vi "niDTS WLAN OFDM Rx Test UTIL OFDM Parameters to WLAN Rx Parameters.vi"(7 "WLAN Rx Input Parameters":T1={"OFDM Data Rate (Mbps)"=enum."6", "Chains"=[TRUE, FALSE, FALSE, FALSE], "Bandwidth (Hz)"=enum."20 MHz", "Channel"=0, "Power (dBm)"=1.0, "16 symbols"=TRUE, "Payload Length (bytes)"=0, "Idle Interval (s)"=7.0, "External Attenuation (dB)"=[0.0, 0.0, 0.0, 0.0], "RX Measurement Parameters"={"Number of Packets"=1000, "MacAddress"="FF:FF:FF:FF:FF:FF"}} {"Idle Interval (s)" format="%_3p"}) -> (8 "WLAN Tx Parameters":T5={"Standard"=enum."802.11 n HT", "DSSS Data Rate (Mbps)"=enum."1", "OFDM Data Rate (Mbps)"=enum."54", "MCS Index"=7, "N Spatial Streams"=1, "Chains"=[TRUE, FALSE, FALSE, FALSE], "Bandwidth (Hz)"=enum."20 MHz", "Channel"=1, "Power (dBm)"=0.0, "Guard Interval"=enum."SHORT", "FEC Coding"=enum."LDPC", "16 symbols"=TRUE, "Payload Length (bytes)"=1500, "Idle Interval (s)"=0.0001, "External Attenuation (dB)"=[0.0, 0.0, 0.0, 0.0], "RX Measurement Parameters"={"Number of Packets"=1000, "MacAddress"="FF:FF:FF:FF:FF:FF"}} {"Idle Interval (s)" format="%_3p"})   [LabVIEW 2014, in "niDTS WLAN.lvlib"]
uses:
  niDTS WLAN.lvlib
  Rx Test/Includes/niDTS WLAN Rx Test INC Parameters.ctl
  Includes/niDTS WLAN INC Standard.ctl
  Includes/niDTS WLAN INC DSSS Data Rate.ctl
  Includes/niDTS WLAN INC OFDM Data Rate.ctl
  Includes/niDTS WLAN INC CH BW.ctl
  Includes/niDTS WLAN INC GI.ctl
  Includes/niDTS WLAN INC FEC Coding.ctl
  Rx Test/Includes/niDTS WLAN INC RX Measurement Parameters.ctl
  Includes/niDTS WLAN Rx Test INC OFDM Parameters.ctl
  Includes/niDTS WLAN INC CH BW DSSS.ctl
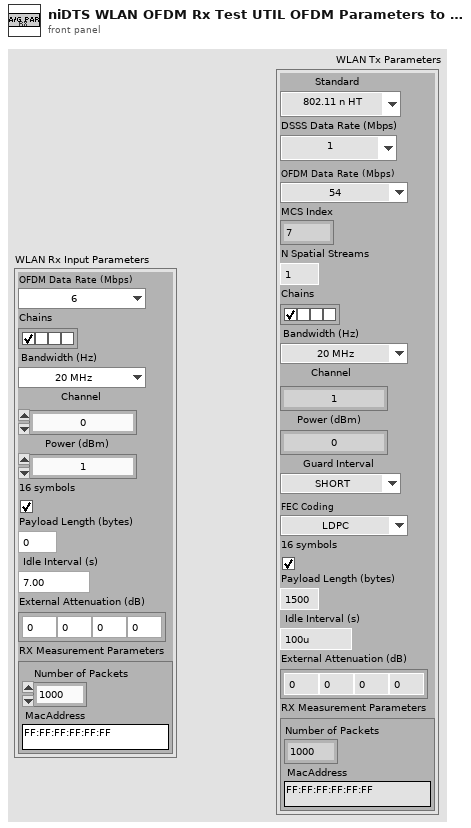
[diagram p1: front panel]
types:
  T1 = typedef "niDTS WLAN.lvlib/niDTS WLAN Rx Test INC OFDM Parameters.ctl" = cluster{"OFDM Data Rate (Mbps)":T2, "Chains":bool[], "Bandwidth (Hz)":T3, "Channel":i32, "Power (dBm)":dbl, "16 symbols":bool, "Payload Length (bytes)":i32, "Idle Interval (s)":dbl, "External Attenuation (dB)":dbl[], "RX Measurement Parameters":T4}
  T2 = typedef "niDTS WLAN.lvlib/niDTS WLAN INC OFDM Data Rate.ctl" = enum16{"6", "9", "12", "18", "24", "36", "48", "54"}
  T3 = typedef "niDTS WLAN.lvlib/niDTS WLAN INC CH BW DSSS.ctl" = enum16{"20 MHz"}
  T4 = typedef "niDTS WLAN.lvlib/niDTS WLAN INC RX Measurement Parameters.ctl" = cluster{"Number of Packets":i32, "MacAddress":string}
  T5 = typedef "niDTS WLAN.lvlib/niDTS WLAN Rx Test INC Parameters.ctl" = cluster{"Standard":T6, "DSSS Data Rate (Mbps)":T7, "OFDM Data Rate (Mbps)":T2, "MCS Index":i32, "N Spatial Streams":i32, "Chains":bool[], "Bandwidth (Hz)":T8, "Channel":i32, "Power (dBm)":dbl, "Guard Interval":T9, "FEC Coding":T10, "16 symbols":bool, "Payload Length (bytes)":i32, "Idle Interval (s)":dbl, "External Attenuation (dB)":dbl[], "RX Measurement Parameters":T4}
  T6 = typedef "niDTS WLAN.lvlib/niDTS WLAN INC Standard.ctl" = enum16{"802.11 b DSSS", "802.11 a/g OFDM", "802.11 n HT", "802.11 ac VHT"}
  T7 = typedef "niDTS WLAN.lvlib/niDTS WLAN INC DSSS Data Rate.ctl" = enum16{"1", "2", "5.5", "11"}
  T8 = typedef "niDTS WLAN.lvlib/niDTS WLAN INC CH BW.ctl" = enum16{"20 MHz", "40 MHz", "80 MHz", "160 MHz"}
  T9 = typedef "niDTS WLAN.lvlib/niDTS WLAN INC GI.ctl" = enum16{"LONG", "SHORT"}
  T10 = typedef "niDTS WLAN.lvlib/niDTS WLAN INC FEC Coding.ctl" = enum16{"BCC", "LDPC"}
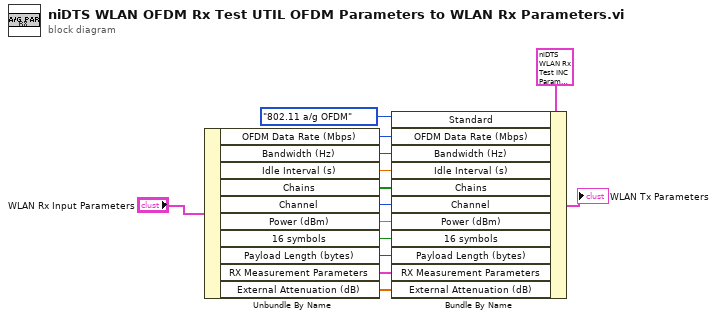
[diagram p0: block diagram]
diagram:
  n1 = Unbundle By Name("WLAN Rx Input Parameters") -> ("OFDM Data Rate (Mbps)"=w11:T2, "Bandwidth (Hz)"=w10:T3, "Idle Interval (s)"=w9:dbl, "Chains"=w8:bool[], "Channel"=w7:i32, "Power (dBm)"=w6:dbl, "16 symbols"=w5:bool, "Payload Length (bytes)"=w4:i32, "RX Measurement Parameters"=w3:T4, "External Attenuation (dB)"=w1:dbl[])
  n2 = Bundle By Name(cluster=T5 {"Standard"=enum."802.11 n HT", "DSSS Data Rate (Mbps)"=enum."1", "OFDM Data Rate (Mbps)"=enum."54", "MCS Index"=7, "N Spatial Streams"=1, "Chains"=[TRUE, FALSE, FALSE, FALSE], "Bandwidth (Hz)"=enum."20 MHz", "Channel"=1, "Power (dBm)"=0.0, "Guard Interval"=enum."SHORT", "FEC Coding"=enum."LDPC", "16 symbols"=TRUE, "Payload Length (bytes)"=1500, "Idle Interval (s)"=0.0001, "External Attenuation (dB)"=[0.0, 0.0, 0.0, 0.0], "RX Measurement Parameters"={"Number of Packets"=1000, "MacAddress"="FF:FF:FF:FF:FF:FF"}} ("WLAN Rx Input Parameters"), "Standard"=niDTS_WLAN_INC_Standard."802.11 a/g OFDM", "OFDM Data Rate (Mbps)"=w11, "Bandwidth (Hz)"=w10, "Idle Interval (s)"=w9, "Chains"=w8, "Channel"=w7, "Power (dBm)"=w6, "16 symbols"=w5, "Payload Length (bytes)"=w4, "RX Measurement Parameters"=w3, "External Attenuation (dB)"=w1) -> (→"WLAN Tx Parameters":T5)
